vi "ProdaNG.Example.GetSystems.vi"() -> ()   [LabVIEW 2016]
panel:
  out "Systems":string[](array[string])
  in  "Connection string":string="prodang/wabco@WPLEXT"
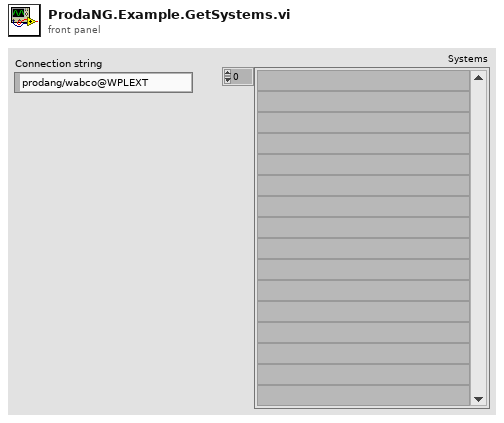
[diagram p1: front panel]
types:
  T1 = typedef "ProdaNG.System.ctl" = cluster{"i_id":i32, "description":string}
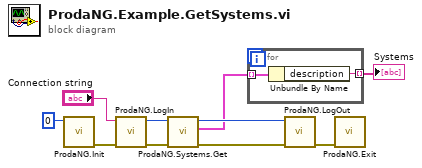
[diagram p0: block diagram]
diagram:
  n1 = call "ProdaNG.Init.vi"("numContexts (0: unlimited)"=0 ("numContexts")) -> ("error out"=w10:errorcluster)  [unwired: 10 in]
  n2 = call "ProdaNG.LogIn.vi"("error in"=w10, "ConnectionString"="Connection string") -> ("error out"=w6:errorcluster, "dbHandle"=w5:i32)  [unwired: 7 in, 1 out]
  n3 = call "ProdaNG.Systems.Get.vi"("error in (no error)"=w6, "dbHandleIn"=w5) -> ("error out"=w4:errorcluster, "Systems"=w2:T1[], "dbHandle"=w3:i32)  [unwired: 7 in]
  n4 = for {
    tunnel: w2 -> [w12] mode=indexing
    tunnel: [w11] -> w1 mode=indexing
    n5 = Unbundle By Name(w12) -> ("description"=w11:string)
  }
  "Systems" <- w1
  n6 = call "ProdaNG.LogOut.vi"("error in"=w4, "dbHandleIn"=w3) -> ("error out"=w8:errorcluster)  [unwired: 9 in]
  n7 = call "ProdaNG.Exit.vi"("error in (no error)"=w8) -> ()  [unwired: 10 in, 1 out]
